vi "MGCC_PV_Fcst_Timer.vi"() -> ()   [LabVIEW 2016]
panel:
  in  "to UTC (F)":bool
  out "hour":i32
  out "minute":i32
  out "second":i32
  in  "want seconds? (F)":bool
  in  "date format (0)":enum16{"short", "long", "abbreviated"}(ring)
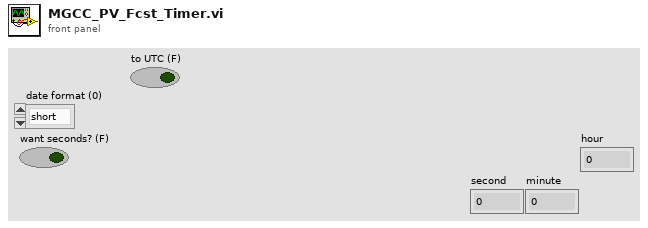
[diagram p1: front panel]
types:
  T1 = typedef "LVDateTimeRec.ctl" = cluster{"fractional second":dbl, "second":i32, "minute":i32, "hour":i32, "day of month":i32, "month":i32, "year":i32, "day of week":i32, "day of year":i32, "DST":i32}
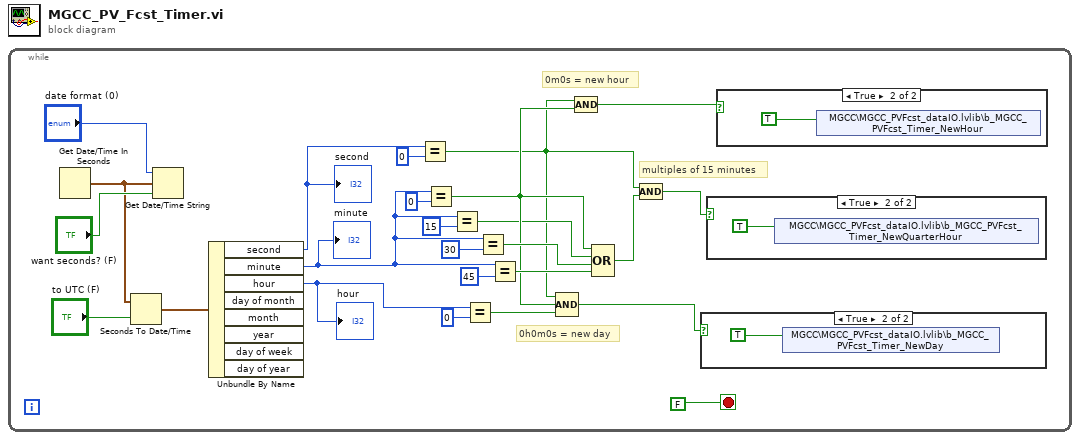
[diagram p0: block diagram]
diagram:
  n1 = while {
    stop <- FALSE ("stop") stop-if-true
    # "multiples of 15 minutes"
    # "0m0s = new hour"
    # "0h0m0s = new day"
    n2 = Get Date/Time In Seconds() -> (seconds since 1Jan1904=w23:timestamp)
    n3 = Seconds To Date/Time(time stamp (now)=w23, to UTC (F)="to UTC (F)") -> (date time rec=w21:T1)
    n4 = Get Date/Time String(date format (0)="date format (0)", seconds (now)=w23, want seconds? (F)="want seconds? (F)") -> ()  [unwired: 2 out]
    n5 = Unbundle By Name(w21) -> ("second"=w19:i32, "minute"=w13:i32, "hour"=w11:i32)  [unwired: 5 out]
    "second" <- w19
    "minute" <- w13
    "hour" <- w11
    n6 = Equal?(x=w19, y=0) -> (x = y?=w4:bool)
    n7 = Equal?(x=w13, y=0) -> (x = y?=w7:bool)
    n8 = Equal?(x=w13, y=15) -> (x = y?=w6:bool)
    n9 = Equal?(x=w11, y=0) -> (x = y?=w10:bool)
    n10 = Equal?(x=w13, y=30) -> (x = y?=w8:bool)
    n11 = Equal?(x=w13, y=45) -> (x = y?=w9:bool)
    n12 = Compound Arithmetic op=AND(w4, w7, w10) -> (w3:bool)
    n13 = Compound Arithmetic op=AND(w4, w7) -> (w1:bool)
    n14 = Compound Arithmetic op=OR(w7, w6, w8, w9) -> (w5:bool)
    n15 = Compound Arithmetic op=AND(w4, w5) -> (w2:bool)
    n16 = case shown="True" w3 {
      frame False {
      }
      frame True {
        n17 = shared-variable "MGCC\\MGCC_PVFcst_dataIO.lvlib\\b_MGCC_PVFcst_Timer_NewDay"(TRUE) -> ()  [unwired: 1 in, 1 out]
      }
    }
    n18 = case shown="True" w2 {
      frame False {
      }
      frame True {
        n19 = shared-variable "MGCC\\MGCC_PVFcst_dataIO.lvlib\\b_MGCC_PVFcst_Timer_NewQuarterHour"(TRUE) -> ()  [unwired: 1 in, 1 out]
      }
    }
    n20 = case shown="True" w1 {
      frame False {
      }
      frame True {
        n21 = shared-variable "MGCC\\MGCC_PVFcst_dataIO.lvlib\\b_MGCC_PVFcst_Timer_NewHour"(TRUE) -> ()  [unwired: 1 in, 1 out]
      }
    }
  }
